vi "removeIDs.vi"(8 "error in (no error)":errorcluster, 10 "IDs":u32[](array[numeric]), 11 "Structure in":refnum<class "Structure.lvclass">) -> (0 "error out":errorcluster, 3 "Structure out":refnum<class "Structure.lvclass">)   [LabVIEW 2009, in "Structure.lvclass"]
uses:
  Structure.lvclass
  Structure.lvclass/Structure.ctl
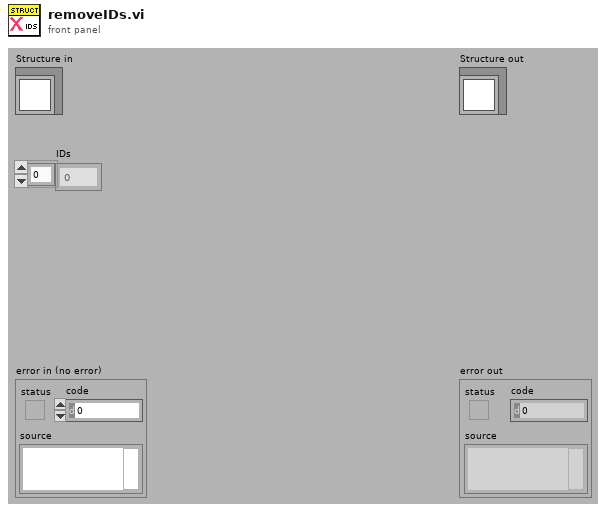
[diagram p1: front panel]
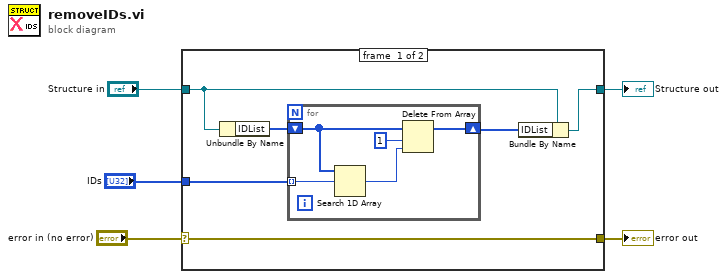
[diagram p0: block diagram]
diagram:
  n1 = case shown="No Error" "error in (no error)" {
    selector: "error in (no error)" -> [w11 w18]
    tunnel: [w11 w18] -> w4
    tunnel: [w6 w17] -> w2
    tunnel: "Structure in" -> [w7 w17]
    tunnel: "IDs" -> [w9 _]
    frame #0 {
      n2 = Unbundle By Name(w7) -> ("IDList"=w10:u32[])
      n3 = for {
        shift-right: [w12] -> w8
        shift-left: w10 -> [w13]
        tunnel: w9 -> [w16] mode=indexing
        n4 = Search 1D Array(1D array=w13, element=w16) -> (index of element=w15:i32)  [unwired: 1 in]
        n5 = Delete From Array(array=w13, length=1, index=w15) -> (array with subset deleted=w12:u32[])  [unwired: 1 out]
      }
      n6 = Bundle By Name(cluster=w7, "IDList"=w8) -> (w6:refnum<class "Structure.lvclass">)
    }
    frame #1 {
    }
  }
  "error out" <- w4
  "Structure out" <- w2
